vi "Configure Load Trigger List.vi"(6 "Delay (0)":i32, 7 "Buffer Name (0: defbuffer1)":i32(ring) items=["defbuffer1", "defbuffer2"], 8 "error in (no error)":errorcluster, 9 "ConfigList (MEASURE_LIST)":string="MEASURE_LIST", 10 "Templates (0: ConfigList)":i32(ring) items=["ConfigList", "Empty"], 11 "VISA resource name":refnum<visa-resource-name>) -> (0 "error out":errorcluster, 3 "VISA resource name out":refnum<visa-resource-name>)   [LabVIEW 2023, in "Keithley DMM6500 DAQ6500 Series.lvlib"]
doc: "Load the trigger config list and empty with the arguments."
uses:
  <instrlib>/Keithley DMM6500 DAQ6500 Series/Keithley DMM6500 DAQ6500 Series.lvlib
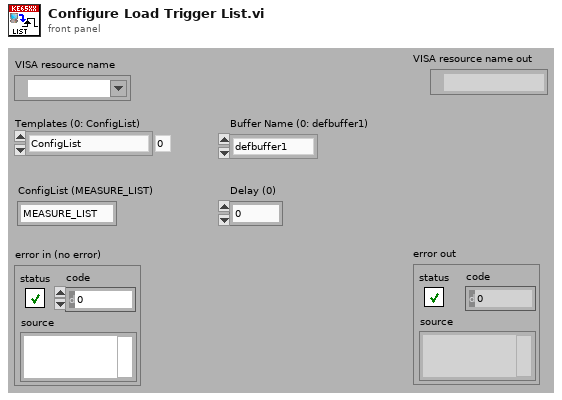
[diagram p1: front panel]
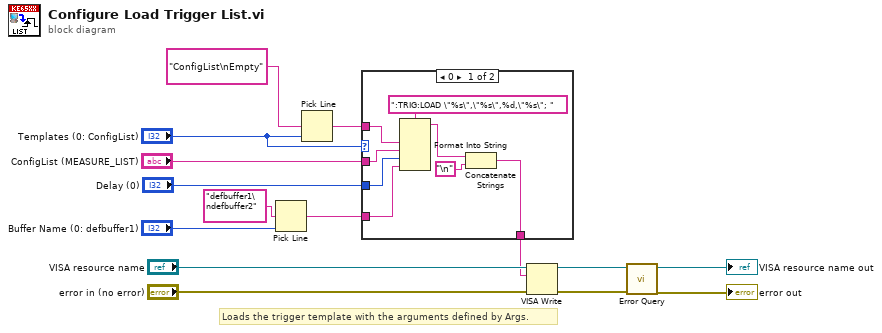
[diagram p0: block diagram]
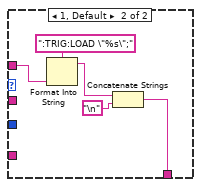
[diagram p2: hidden frame]
diagram:
  # "Loads the trigger template with the arguments defined by Args."
  n1 = Pick Line(multi-line string="defbuffer1\ndefbuffer2", line index="Buffer Name (0: defbuffer1)") -> (output string=w1:string)  [unwired: 1 in]
  n2 = Pick Line(multi-line string="ConfigList\nEmpty", line index="Templates (0: ConfigList)") -> (output string=w9:string)  [unwired: 1 in]
  n3 = case shown="0" "Templates (0: ConfigList)" {
    tunnel: w9 -> [w22 w27]
    tunnel: [w21 w26] -> w7
    tunnel: "ConfigList (MEASURE_LIST)" -> [w18 _]
    tunnel: "Delay (0)" -> [w17 _]
    tunnel: w1 -> [w16 _]
    frame 0 {
      n4 = Format Into String(format string=":TRIG:LOAD \"%s\",\"%s\",%d,\"%s\"; ", w22, w18, w17, w16) -> (resulting string=w20:string)  [unwired: 2 in, 1 out]
      n5 = Concatenate Strings(w20, "\n") -> (w21:string)
    }
    frame 1, Default {
      n6 = Format Into String(format string=":TRIG:LOAD \"%s\";", w27) -> (resulting string=w25:string)  [unwired: 2 in, 1 out]
      n7 = Concatenate Strings(w25, "\n") -> (w26:string)
    }
  }
  n8 = VISA Write(VISA resource name="VISA resource name", write buffer=w7, error in (no error)="error in (no error)") -> (VISA resource name out=w13:refnum<visa-resource-name>, error out=w12:errorcluster)  [unwired: 1 out]
  n9 = call <instrlib>:"Error Query.vi"("error in (no error)"=w12, "VISA resource name"=w13) -> ("error out"=→"error out":errorcluster, "VISA resource name out"=→"VISA resource name out":refnum<visa-resource-name>)  [unwired: 6 in, 2 out]
